vi "Todo1.vi"() -> ()   [LabVIEW 2020]
panel:
  in  "Reset":bool
  in  "stop":bool
  out "led0":bool
  out "led1":bool
  out "led2":bool
  out "led3":bool
  in  "Count up by 2":bool
  in  "Count up By 1":bool
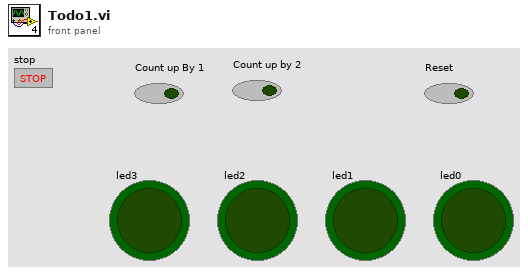
[diagram p1: front panel]
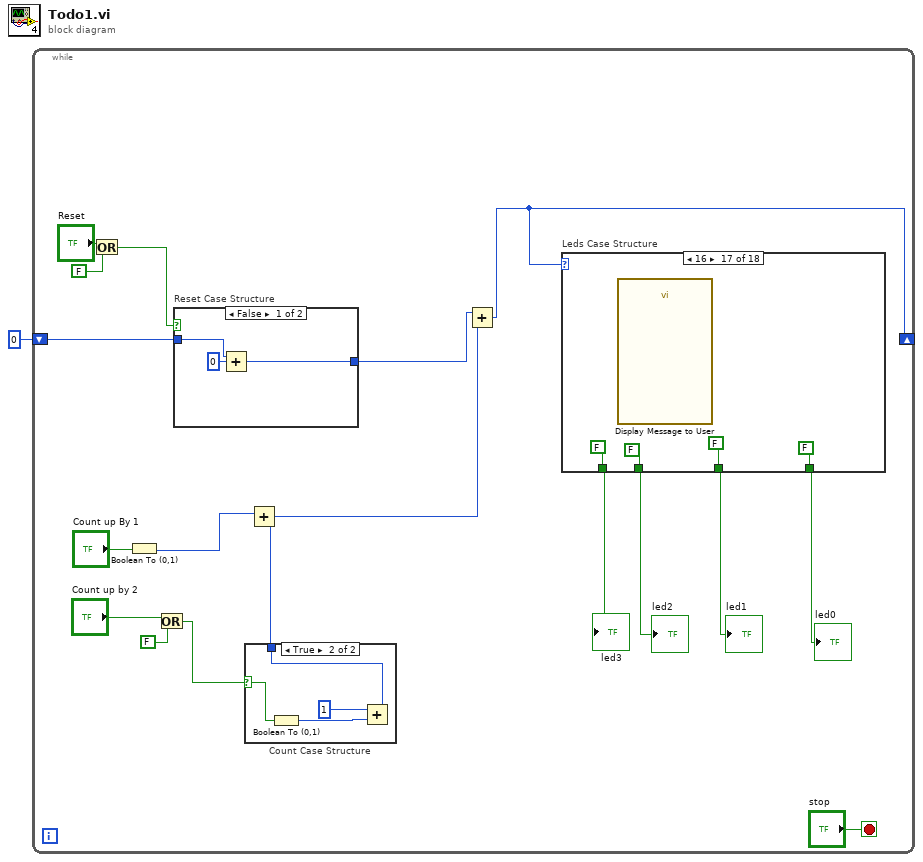
[diagram p0: block diagram]
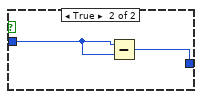
[diagram p2: hidden frame]
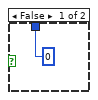
[diagram p3: hidden frame]
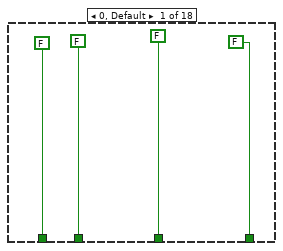
[diagram p4: hidden frame]
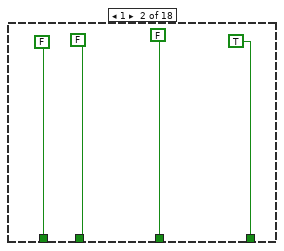
[diagram p5: hidden frame]
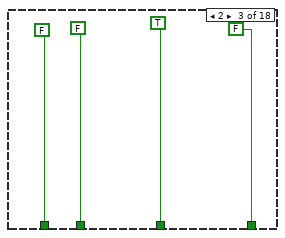
[diagram p6: hidden frame]
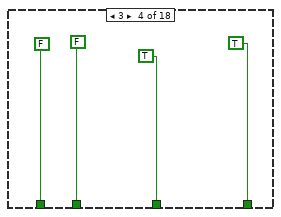
[diagram p7: hidden frame]
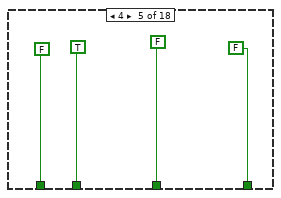
[diagram p8: hidden frame]
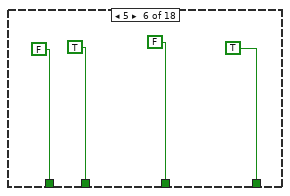
[diagram p9: hidden frame]
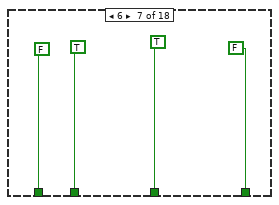
[diagram p10: hidden frame]
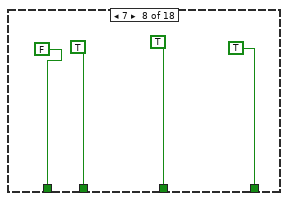
[diagram p11: hidden frame]
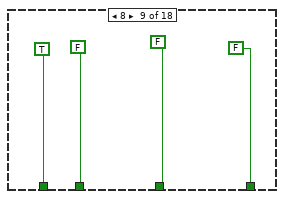
[diagram p12: hidden frame]
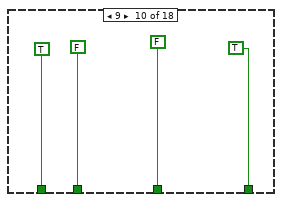
[diagram p13: hidden frame]
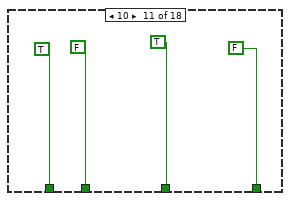
[diagram p14: hidden frame]
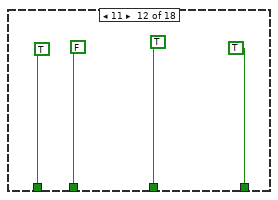
[diagram p15: hidden frame]
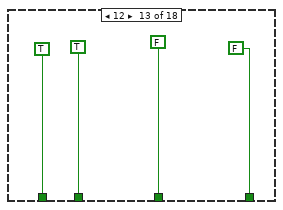
[diagram p16: hidden frame]
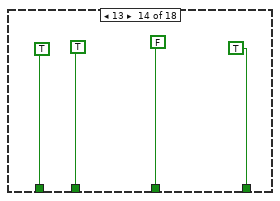
[diagram p17: hidden frame]
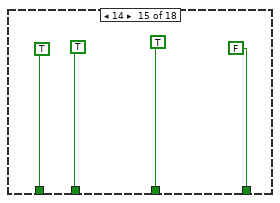
[diagram p18: hidden frame]
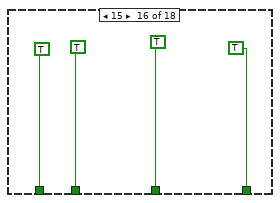
[diagram p19: hidden frame]
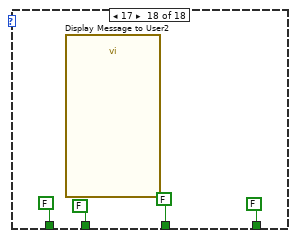
[diagram p20: hidden frame]
diagram:
  n1 = while {
    shift-right: [w18] -> _
    shift-left: 0 -> [w4]
    stop <- "stop" stop-if-true
    n2 = Or(x="Reset", y=FALSE ("x .or. y?")) -> (x .or. y?=w2:bool)
    n3 = Boolean To (0,1)(Boolean="Count up By 1") -> (0, 1=w11:i16)
    n4 = Or(x="Count up by 2", y=FALSE ("x .or. y?")) -> (x .or. y?=w8:bool)
    n5 = case "Reset Case Structure" shown="False" w2 {
      tunnel: w4 -> [w22 w24]
      tunnel: [w20 w23] -> w3
      frame False {
        n6 = Add(x=w22, y=0 ("x+y")) -> (x+y=w20:i32)
      }
      frame True {
        n7 = Subtract(x=w24, y=w24) -> (x-y=w23:i32)
      }
    }
    n8 = case "Count Case Structure" shown="True" w8 {
      selector: w8 -> [_ w29]
      tunnel: [i16 0 ("y") w26] -> w10
      frame False {
      }
      frame True {
        n9 = Boolean To (0,1)(Boolean=w29) -> (0, 1=w28:i16)
        n10 = Add(x=i16 1 ("y"), y=w28) -> (x+y=w26:i16)
      }
    }
    n11 = Add(x=w11, y=w10) -> (x+y=w5:i16)
    n12 = Add(x=w3, y=w5) -> (x+y=w18:i32)
    n13 = case "Leds Case Structure" shown="16" w18 {
      tunnel: [FALSE ("led0") FALSE ("led0") TRUE ("led0") TRUE ("led0") FALSE ("led0") FALSE ("led0") TRUE ("led0") TRUE ("led0") FALSE ("led0") FALSE ("led0") TRUE ("led0") TRUE ("led0") FALSE ("led0") FALSE ("led0") TRUE ("led0") TRUE ("led0") FALSE FALSE] -> w17
      tunnel: [FALSE ("led0") FALSE ("led0") FALSE ("led0") FALSE ("led0") TRUE ("led0") TRUE ("led0") TRUE ("led0") TRUE ("led0") FALSE ("led0") FALSE ("led0") FALSE ("led0") FALSE ("led0") TRUE ("led0") TRUE ("led0") TRUE ("led0") TRUE ("led0") FALSE FALSE] -> w16
      tunnel: [FALSE ("led0") FALSE ("led0") FALSE ("led0") FALSE ("led0") FALSE ("led0") FALSE ("led0") FALSE ("led0") FALSE ("led0") TRUE ("led0") TRUE ("led0") TRUE ("led0") TRUE ("led0") TRUE ("led0") TRUE ("led0") TRUE ("led0") TRUE ("led0") FALSE FALSE] -> w15
      tunnel: [FALSE ("led0") TRUE ("led0") FALSE ("led0") TRUE ("led0") FALSE ("led0") TRUE ("led0") FALSE ("led0") TRUE ("led0") FALSE ("led0") TRUE ("led0") FALSE ("led0") TRUE ("led0") FALSE ("led0") TRUE ("led0") FALSE ("led0") TRUE ("led0") FALSE FALSE] -> w14
      frame 0, Default {
      }
      frame 1 {
      }
      frame 2 {
      }
      frame 3 {
      }
      frame 4 {
      }
      frame 5 {
      }
      frame 6 {
      }
      frame 7 {
      }
      frame 8 {
      }
      frame 9 {
      }
      frame 10 {
      }
      frame 11 {
      }
      frame 12 {
      }
      frame 13 {
      }
      frame 14 {
      }
      frame 15 {
      }
      frame 16 {
        n14 = call "Display Message to User"() -> ()  [unwired: 10 in, 2 out]
      }
      frame 17 {
        n15 = call "Display Message to User2"() -> ()  [unwired: 10 in, 2 out]
      }
    }
    "led0" <- w14
    "led1" <- w17
    "led2" <- w16
    "led3" <- w15
  }
